vi "PFI-28000-Overload_Get Overload.vi"(8 "error in (no error)":errorcluster, 11 "PFI-28000-Overload in":refnum<class "PFI-28000-Overload.lvclass">) -> (0 "error out":errorcluster, 2 "Overload":T1, 3 "PFI-28000-Overload out":refnum<class "PFI-28000-Overload.lvclass">)   [LabVIEW 2017, in "PFI-28000-Overload.lvclass"]
uses:
  PFI-28000-Overload.lvclass
  PFI-28000-Overload-Type.ctl
  PFI-28000-Overload.lvclass/PFI-28000-Overload.ctl
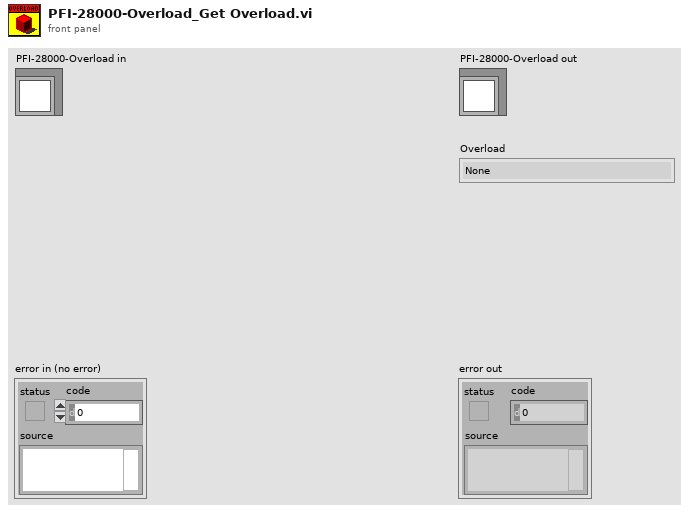
[diagram p1: front panel]
types:
  T1 = typedef "PFI-28000-Overload.lvclass/PFI-28000-Overload-Type.ctl" = enum8{"None", "Filter Input", "Input", "Output", "Open", "Short", "Alarm"}
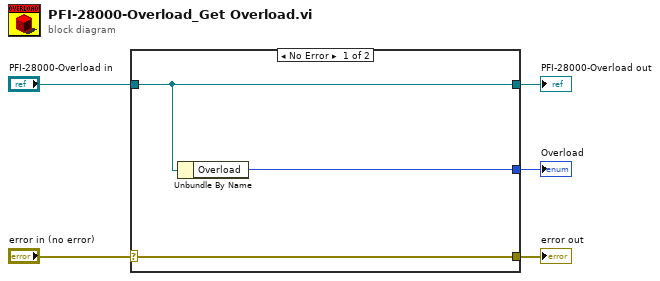
[diagram p0: block diagram]
diagram:
  n1 = case shown="No Error" "error in (no error)" {
    selector: "error in (no error)" -> [w8 w9]
    tunnel: [w8 w9] -> w4
    tunnel: [w7 w10] -> w2
    tunnel: "PFI-28000-Overload in" -> [w7 w10]
    tunnel: [w6 _] -> w1
    frame No Error {
      n2 = Unbundle By Name(w7) -> ("Overload"=w6:T1)
    }
    frame Error {
    }
  }
  "error out" <- w4
  "PFI-28000-Overload out" <- w2
  "Overload" <- w1
